vi "example_02_pagination_controls.vi"() -> ()   [LabVIEW 2015, in "lv-pagination.lvlib"]
doc: "This example shows how you can change the data for a static set of controls using scrollbars simlar to example 01."
uses:
  lv-pagination.lvlib
panel:
  out "data [[]]":dbl[][](array[numeric])
  in  "scrollbar_horizontal":i32(c297)
  in  "columns":i32=4
  in  "rows":i32=100
  in  "scrollbar_vertical":i32(c297)
  in  "number_4_4":dbl
  in  "number_3_4":dbl
  in  "number_2_4":dbl
  in  "number_1_4":dbl
  in  "number_4_3":dbl
  in  "number_3_3":dbl
  in  "number_2_3":dbl
  in  "number_1_3":dbl
  in  "number_4_2":dbl
  in  "number_3_2":dbl
  in  "number_2_2":dbl
  in  "number_1_2":dbl
  in  "number_4_1":dbl
  in  "number_3_1":dbl
  in  "number_2_1":dbl
  in  "number_1_1":dbl
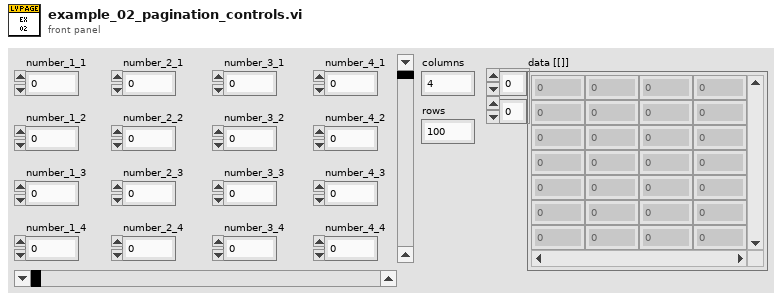
[diagram p1: front panel]
types:
  T1 = enum8{"Enabled", "Disabled", "Disabled and Grayed Out"}
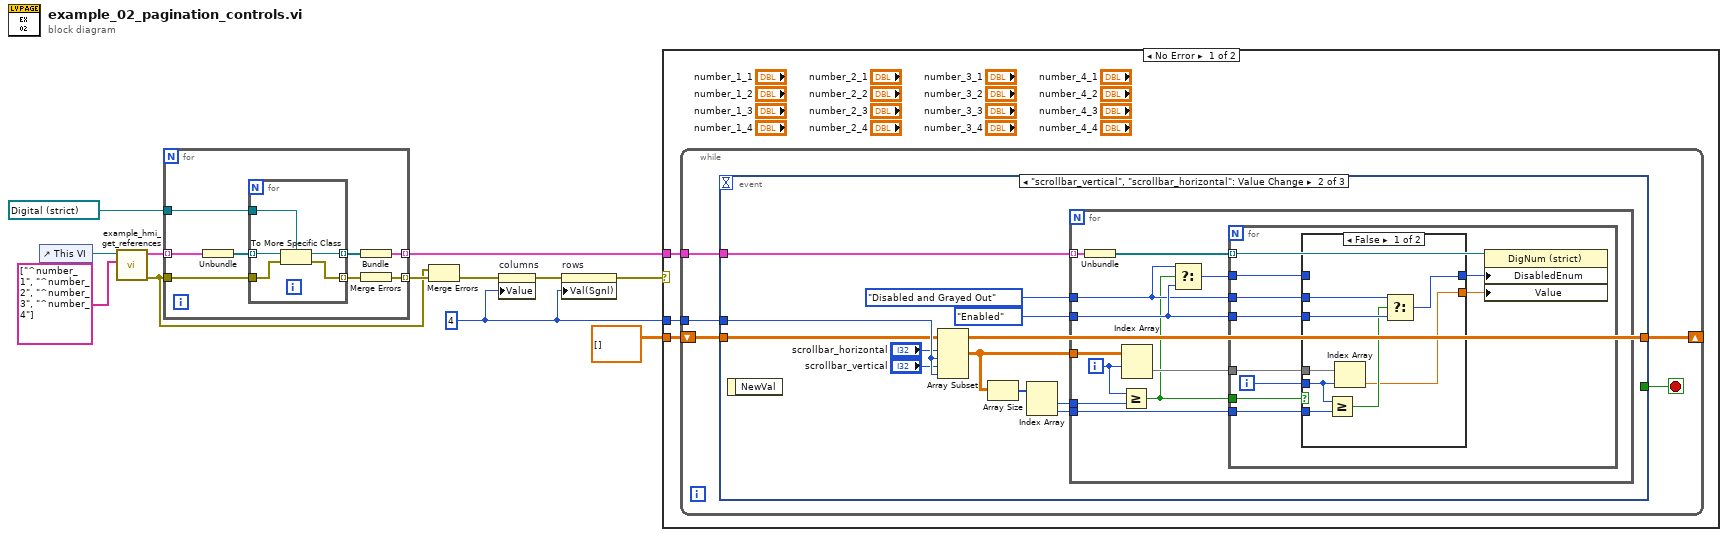
[diagram p0: block diagram]
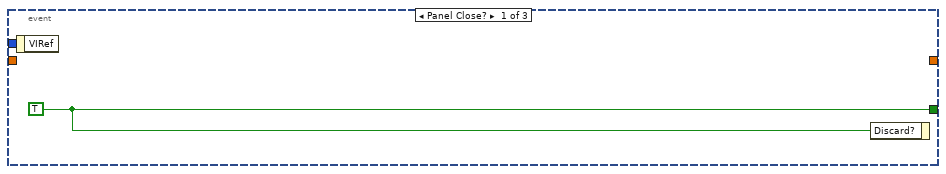
[diagram p2: hidden frame]
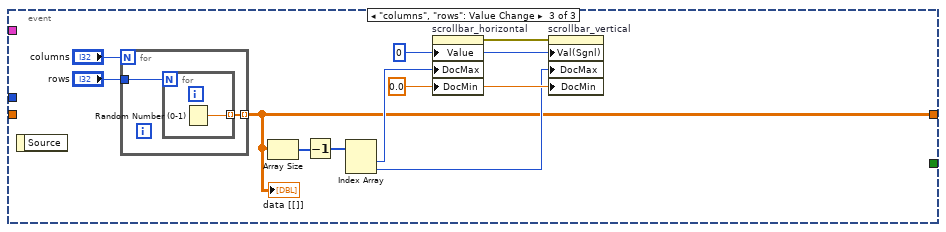
[diagram p4: hidden frame]
diagram:
  w5 = 4 ("y")
  n1 = control-ref of="This VI"() -> (w12:refnum<vi>)
  n2 = call "example_hmi_get_references.vi"("control_search []"=string[] ["^number_1", "^number_2", "^number_3", "^number_4"], "vi_reference"=w12) -> ("error out"=w1:errorcluster, "references"=w11:cluster{refnum<vi>[]}[])  [unwired: 8 in]
  n3 = for {
    tunnel: w11 -> [w20] mode=indexing
    tunnel: refnum<vi> refnum ("number_1_1") -> [w18]
    tunnel: w1 -> [w17]
    tunnel: [w15] -> w8 mode=indexing
    tunnel: [w14] -> w9 mode=indexing
    n4 = Unbundle(w20) -> (w19:refnum<vi>[])
    n5 = for {
      tunnel: w19 -> [w25] mode=indexing
      tunnel: w18 -> [w24]
      tunnel: w17 -> [w23]
      tunnel: [w22] -> w16 mode=indexing
      tunnel: [w21] -> w13 mode=indexing
      n6 = To More Specific Class(target class=w24, reference=w25, error in=w23) -> (specific class reference=w22:refnum<vi>, error out=w21:errorcluster)
    }
    n7 = Bundle(w16) -> (w15:cluster{refnum<vi>[]})  [unwired: 1 in]
    n8 = Merge Errors(w13) -> (w14:errorcluster)
  }
  n9 = Merge Errors(w1, w9) -> (w3:errorcluster)
  n10 = property on="columns" class="DigNum (strict)"(error in=w3, "Value"=w5) -> (error out=w4:errorcluster)  [unwired: 1 in, 1 out]
  n11 = property on="rows" class="DigNum (strict)"(error in=w4, "Val(Sgnl)"=w5) -> (error out=w2:errorcluster)  [unwired: 1 in, 1 out]
  n12 = case shown="No Error" w2 {
    tunnel: w8 -> [w28 _]
    tunnel: dbl[][] [] -> [w27 _]
    tunnel: w5 -> [w26 _]
    frame No Error {
      n13 = while {
        tunnel: w28 -> [w32]
        tunnel: w26 -> [w30]
        shift-right: [w29] -> _
        shift-left: w27 -> [w31]
        stop <- w33 stop-if-true
        n14 = event shown="[1] \"scrollbar_vertical\", \"scrollbar_horizontal\": Value Change" {
          selector: _ -> [_ _ _]
          dyn-events: _ -> [_ _ _]
          timeout: _ -> [_ _ _]
          tunnel: [w34 _ _] -> w33
          tunnel: w32 -> [_ w45 _]
          tunnel: w31 -> [_ w35 _]
          tunnel: w30 -> [_ w43 _]
          tunnel: [_ w35 w77] -> w29
          event Panel Close? {
            w34 = TRUE
            n15 = event-data() -> ()  [unwired: 1 in, 1 out]
            n16 = event-data("Discard?"=w34) -> ()  [unwired: 1 in, 1 out]
          }
          event "scrollbar_vertical", "scrollbar_horizontal": Value Change {
            n17 = event-data() -> ()  [unwired: 1 in, 1 out]
            n18 = Array Subset(array=w35, index (row)="scrollbar_horizontal", length (row)=w43, index (col)="scrollbar_vertical", length (col)=w43) -> (w44:dbl[][])
            n19 = Array Size(array=w44) -> (size(s)=w38:i32[])
            n20 = Index Array(array=w38) -> (element #1=w42:i32, element #2=w41:i32)  [unwired: 2 in]
            n21 = for {
              tunnel: w45 -> [w56] mode=indexing
              tunnel: w44 -> [w49]
              tunnel: w42 -> [w53]
              tunnel: w41 -> [w54]
              tunnel: T1."Disabled and Grayed Out" ("Disabled") -> [w51]
              tunnel: T1."Enabled" ("Disabled") -> [w52]
              i -> [w47]
              n22 = Unbundle(w56) -> (w55:refnum<vi>[])
              n23 = Greater Or Equal?(x=w47, y=w53) -> (x >= y?=w46:bool)
              n24 = Index Array(array=w49, index (row)=w47) -> (element=w48:dbl[])  [unwired: 1 in]
              n25 = Select(t=w51, s=w46, f=w52) -> (s? t:f=w50:T1)
              n26 = for {
                tunnel: w55 -> [w66] mode=indexing
                tunnel: w54 -> [w65]
                tunnel: w52 -> [w64]
                tunnel: w51 -> [w63]
                tunnel: w50 -> [w62]
                tunnel: w48 -> [w60]
                tunnel: w46 -> [w57]
                i -> [w58]
                n27 = case shown="False" w57 {
                  tunnel: w65 -> [w74 _]
                  tunnel: w64 -> [w73 _]
                  tunnel: w63 -> [w72 _]
                  tunnel: w62 -> [_ w75]
                  tunnel: [w67 w75] -> w61
                  tunnel: w60 -> [w70 _]
                  tunnel: [w69 _] -> w59
                  tunnel: w58 -> [w68 _]
                  frame False {
                    n28 = Greater Or Equal?(x=w68, y=w74) -> (x >= y?=w71:bool)
                    n29 = Index Array(array=w70, index=w68) -> (element=w69:dbl)
                    n30 = Select(t=w72, s=w71, f=w73) -> (s? t:f=w67:T1)
                  }
                  frame True {
                  }
                }
                n31 = property class="DigNum (strict)"(reference=w66, "DisabledEnum"=w61, "Value"=w59) -> ()  [unwired: 1 in, 2 out]
              }
            }
          }
          event "columns", "rows": Value Change {
            w83 = 0.0 ("Doc Min")
            w80 = 0 ("Value (Signaling)")
            n32 = event-data() -> ()  [unwired: 1 in, 1 out]
            n33 = for {
              N: "columns" -> [_]
              tunnel: [w87] -> w77 mode=indexing
              tunnel: "rows" -> [w86]
              n34 = for {
                N: w86 -> [_]
                tunnel: [w88] -> w87 mode=indexing
                n35 = Random Number (0-1)() -> (number: 0 to 1=w88:dbl)
              }
            }
            "data [[]]" <- w77
            n36 = Array Size(array=w77) -> (size(s)=w78:i32[])
            n37 = Decrement(x=w78) -> (x-1=w76:i32[])
            n38 = Index Array(array=w76) -> (element #1=w81:i32, element #2=w79:i32)  [unwired: 2 in]
            n39 = property on="scrollbar_horizontal" class="Scroll (strict)"("Value"=w80, "DocMax"=w81, "DocMin"=w83) -> (error out=w82:errorcluster)  [unwired: 2 in, 1 out]
            n40 = property on="scrollbar_vertical" class="Scroll (strict)"(error in=w82, "Val(Sgnl)"=w80, "DocMax"=w79, "DocMin"=w83) -> ()  [unwired: 1 in, 2 out]
          }
        }
      }
    }
    frame Error {
    }
  }
